vi "Get SV Host.vi"(11 "AEgIS Shared Variables in":refnum<class "Circus Shared Variables.lvclass">) -> (2 "Host":string, 3 "AEgIS Shared Variables out":refnum<class "Circus Shared Variables.lvclass">)   [LabVIEW 2026, in "TALOS.lvlib" / "Classes.lvlib" / "Circus Shared Variables.lvclass"]
uses:
  Circus Shared Variables.lvclass
  Circus Shared Variables.lvclass/Circus Shared Variables.ctl
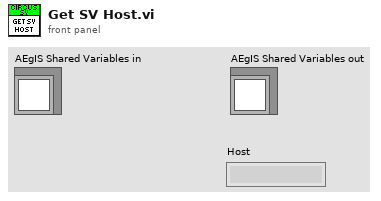
[diagram p1: front panel]
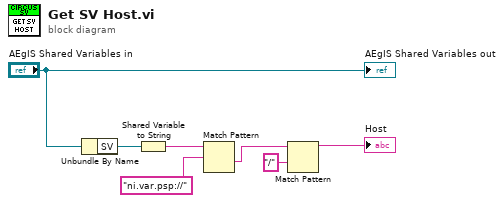
[diagram p0: block diagram]
diagram:
  n1 = Unbundle By Name("AEgIS Shared Variables in") -> ("SV"=w5:refnum<k21>)
  n2 = Shared Variable to String(1:w5) -> (0:w4:string)
  n3 = Match Pattern(string=w4, regular expression="ni.var.psp://") -> (after substring=w2:string)  [unwired: 1 in, 3 out]
  n4 = Match Pattern(string=w2, regular expression="/") -> (before substring=→"Host":string)  [unwired: 1 in, 3 out]
  "AEgIS Shared Variables out" <- "AEgIS Shared Variables in"
